vi "IP Address Facade.vi"(0 "Data In":T4="0.0.0.0", 2 "Display State In":T2, 3 "Container State":T3) -> (6 "Data Out":T4="0.0.0.0", 7 "Display State Out":T2, 8 "Action":T1)   [LabVIEW 2011, in "IP Address.xctl"]
doc: "The control takes data in the form of 4 individual unsigned bytes and automatically converts to a string representation of an IP address such as 127.0.0.1. An addition to that, the control advances the cursor to the next byte when it detects three characters, the Tab key, or the Period/Dot/Decimal key.\n\nv1.0 Copyright 2007 - Dan Press - PrimeTest Automation"
uses:
  IP Address.xctl
  IP Address Data.ctl
  <vilib>/_xctls/Container State.ctl
  IP Address State.ctl
  <vilib>/_xctls/Action.ctl
  <vilib>/_xctls/XControlSupport.lvlib
panel:
  in  "IP Address (ctl)":T5
  out "IP Address (ind)":T5
  # "."
  # "."
  # "."
  # "."
  # "."
  # "."
  # "."
  # "."
  # "."
  # "."
  # "."
  # "."
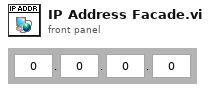
[diagram p1: front panel]
types:
  T1 = typedef "XControlSupport.lvlib/Action.ctl" = cluster{"Data Changed?":bool, "State Changed?":bool, "Action Name":string}
  T2 = typedef "IP Address.xctl/IP Address State.ctl" = cluster{"Byte":i32, "Address":cluster{"IP 0":u8, "IP 1":u8, "IP 2":u8, "IP 3":u8}}
  T3 = typedef "XControlSupport.lvlib/Container State.ctl" = cluster{"Indicator?":bool, "Run Mode?":bool, " Refnum":refnum<vi>}
  T4 = typedef "IP Address.xctl/IP Address Data.ctl" = string
  T5 = cluster{"IP 0":u8, "IP 1":u8, "IP 2":u8, "IP 3":u8}
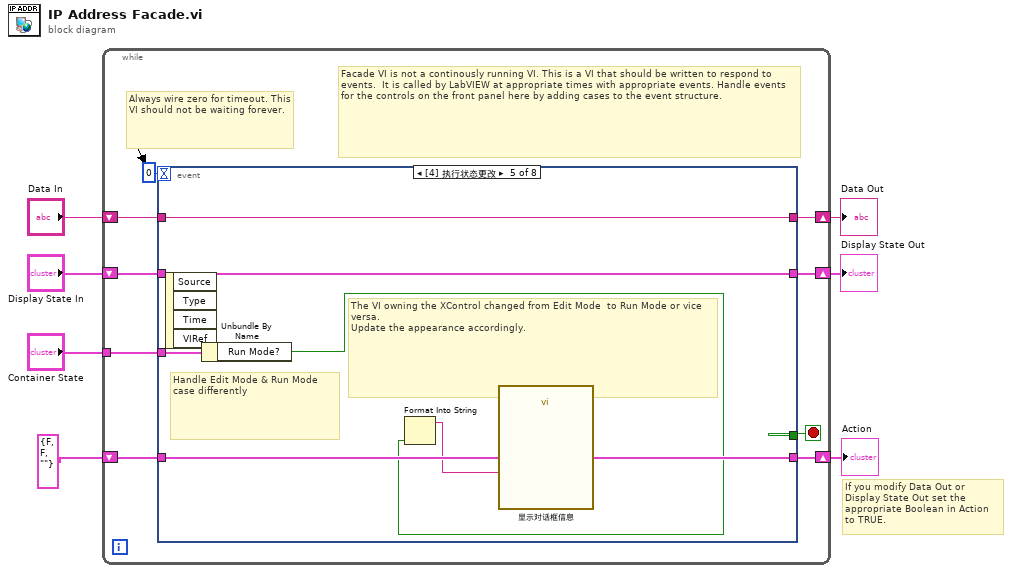
[diagram p0: block diagram]
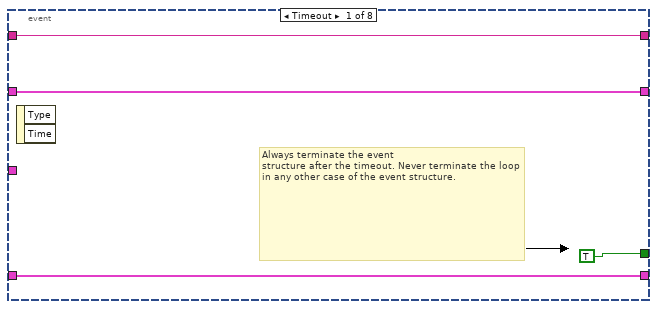
[diagram p2: hidden frame]
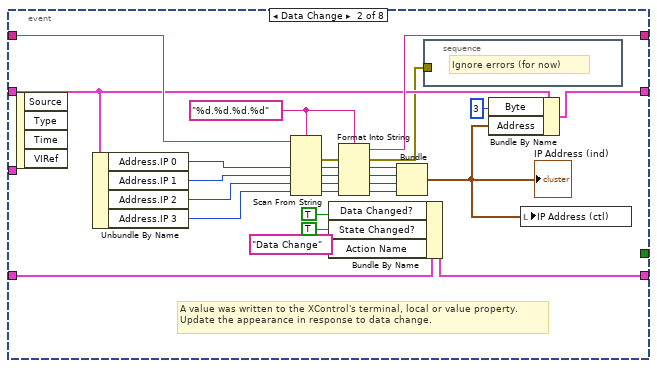
[diagram p3: hidden frame]
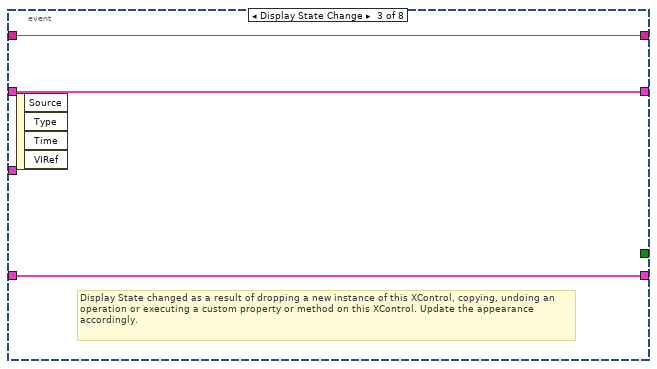
[diagram p4: hidden frame]
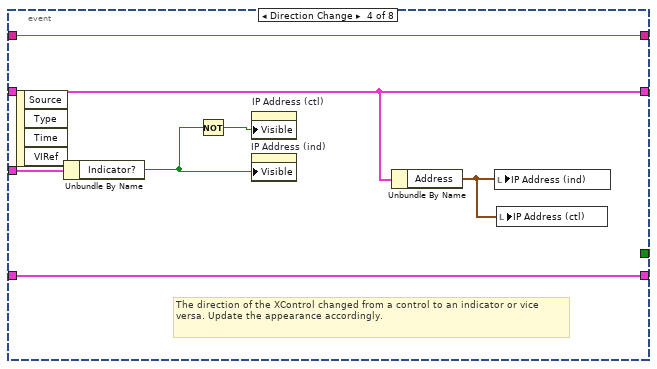
[diagram p5: hidden frame]
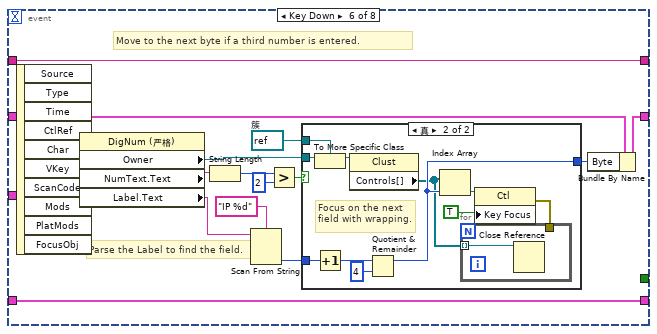
[diagram p6: hidden frame]
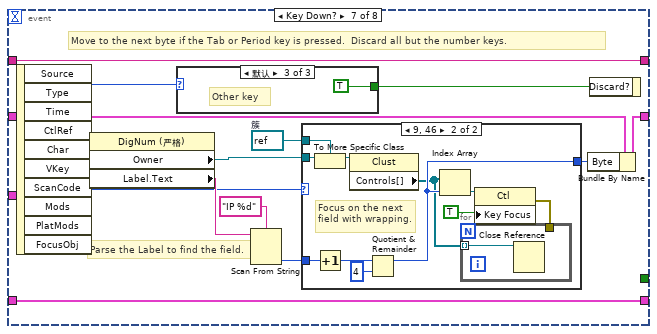
[diagram p8: hidden frame]
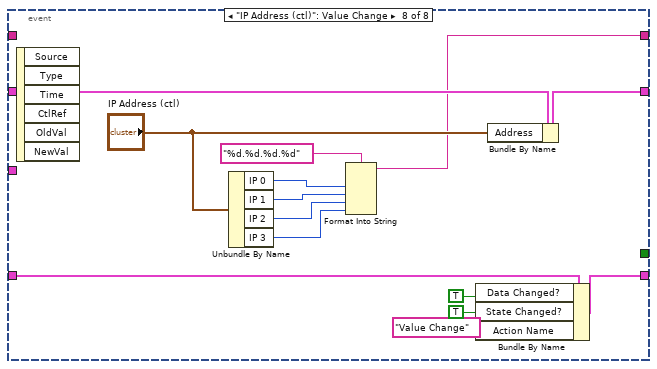
[diagram p12: hidden frame]
diagram:
  # "If you modify Data Out or\nDisplay State Out set the\nappropriate Boolean in Action\nto TRUE."
  n1 = while {
    shift-right: [w15] -> w4
    shift-left: "Display State In" -> [w16]
    tunnel: "Container State" -> [w12]
    shift-right: [w10] -> w7
    shift-left: "Data In" -> [w11]
    shift-right: [w8] -> w2
    shift-left: T1 {"Data Changed?"=FALSE, "State Changed?"=FALSE, "Action Name"=""} ("Action") -> [w9]
    stop <- w14 stop-if-true
    # "Facade VI is not a continously running VI. This is a VI that should be written to respond to events.  It is called by LabVIEW at appropriate times with appropriate events. Handle events for the controls on the front panel here by adding cases to the event structure."
    # "Always wire zero for timeout. This\nVI should not be waiting forever."
    n2 = event shown="[4] 执行状态更改" {
      selector: _ -> [_ _ _ _ _ _ _ _]
      dyn-events: _ -> [_ _ _ _ _ _ _ _]
      timeout: 0 -> [_ _ _ _ _ _ _ _]
      tunnel: w16 -> [w18 w31 w43 w47 w57 w67 w96 w127]
      tunnel: [w18 w30 w43 w47 w57 w66 w95 w126] -> w15
      tunnel: [TRUE _ _ _ _ _ _ _] -> w14
      tunnel: w12 -> [_ _ _ w52 w58 _ _ _]
      tunnel: w11 -> [w17 w33 w45 w51 w56 w73 w99 _]
      tunnel: [w17 w32 w45 w51 w56 w73 w99 w119] -> w10
      tunnel: [w19 w27 w44 w50 w55 w72 w98 w117] -> w8
      tunnel: w9 -> [w19 w28 w44 w50 w55 w72 w98 w118]
      event Timeout {
        # "Always terminate the event\nstructure after the timeout. Never terminate the loop in any other case of the event structure."
        n3 = event-data() -> ()  [unwired: 1 in, 2 out]
      }
      event Data Change {
        w34 = "%d.%d.%d.%d" ("format string")
        # "A value was written to the XControl's terminal, local or value property.\nUpdate the appearance in response to data change."
        n4 = event-data() -> ()  [unwired: 1 in, 4 out]
        n5 = Unbundle By Name(w31) -> ("Address.IP 0"=w42:u8, "Address.IP 1"=w41:u8, "Address.IP 2"=w40:u8, "Address.IP 3"=w39:u8)
        n6 = Scan From String(format string=w34, input string=w33, default 1=w42, default 2=w41, default 3=w40, default 4=w39) -> (error out=w22:errorcluster, output 1=w38:u8, output 2=w37:u8, output 3=w36:u8, output 4=w35:u8)  [unwired: 2 in, 2 out]
        n7 = Bundle By Name(cluster=w28, "Data Changed?"=TRUE, "State Changed?"=TRUE, "Action Name"="Data Change") -> (w27:T1)
        n8 = Format Into String(format string=w34, error in=w22, w38, w37, w36, w35) -> (resulting string=w32:string, error out=w21:errorcluster)  [unwired: 1 in]
        n9 = Bundle("IP 0"=w38, "IP 1"=w37, "IP 2"=w36, "IP 3"=w35) -> (w23:T5)  [unwired: 1 in]
        "IP Address (ind)" <- w23
        n10 = stacked-sequence {
          tunnel: w21 -> [_]
          frame #0 {
            # "Ignore errors (for now)"
          }
        }
        n11 = Bundle By Name(cluster=w31, "Byte"=3, "Address"=w23) -> (w30:T2)
        n12 = local write "IP Address (ctl)"(w23) -> ()
      }
      event Display State Change {
        # "Display State changed as a result of dropping a new instance of this XControl, copying, undoing an operation or executing a custom property or method on this XControl. Update the appearance accordingly."
        n13 = event-data() -> ()  [unwired: 1 in, 4 out]
      }
      event Direction Change {
        # "The direction of the XControl changed from a control to an indicator or vice versa. Update the appearance accordingly."
        n14 = event-data() -> ()  [unwired: 1 in, 4 out]
        n15 = Unbundle By Name(w52) -> ("Indicator?"=w49:bool)
        n16 = Not(x=w49) -> (.not. x?=w48:bool)
        n17 = property on="IP Address (ctl)" class="Clust (严格)"("Visible"=w48) -> ()  [unwired: 2 in, 2 out]
        n18 = property on="IP Address (ind)" class="Clust (严格)"("Visible"=w49) -> ()  [unwired: 2 in, 2 out]
        n19 = Unbundle By Name(w47) -> ("Address"=w46:T5)
        n20 = local write "IP Address (ind)"(w46) -> ()
        n21 = local write "IP Address (ctl)"(w46) -> ()
      }
      event Exec State Change {
        # "The VI owning the XControl changed from Edit Mode  to Run Mode or vice versa.\nUpdate the appearance accordingly."
        # "Handle Edit Mode & Run Mode\ncase differently"
        n22 = event-data() -> ()  [unwired: 1 in, 4 out]
        n23 = Unbundle By Name(w58) -> ("Run Mode?"=w54:bool)
        n24 = Format Into String(w54) -> (resulting string=w53:string)  [unwired: 3 in, 1 out]
        n25 = call "显示对话框信息"("Message"=w53) -> ()  [unwired: 9 in, 2 out]
      }
      event "IP Address (ctl).IP 0", "IP Address (ctl).IP 1", "IP Address (ctl).IP 2", "IP Address (ctl).IP 3": Key Down {
        w59 = refnum<vi> refnum  # 簇
        # "Move to the next byte if a third number is entered."
        # "Parse the Label to find the field."
        n26 = event-data() -> ("CtlRef"=w71:refnum<vi>)  [unwired: 1 in, 9 out]
        n27 = property class="DigNum (严格)"(reference=w71) -> ("Owner"=w60:refnum<vi>, "NumText.Text"=w70:string, "Label.Text"=w65:string)  [unwired: 1 in, 2 out]
        n28 = String Length(string=w70) -> (length=w69:i32)
        n29 = Scan From String(format string="IP %d", input string=w65) -> (output 1=w62:i32)  [unwired: 3 in, 3 out]
        n30 = Greater?(x=w69, y=2) -> (0:w63:bool)
        n31 = case shown="真" w63 {
          tunnel: w62 -> [w74 w85]
          tunnel: [w74 w79] -> w61
          tunnel: w60 -> [_ w82]
          tunnel: w59 -> [_ w80]
          frame False {
          }
          frame True {
            # "Focus on the next field with wrapping."
            n32 = To More Specific Class(target class=w80, reference=w82) -> (specific class reference=w81:refnum<vi>)  [unwired: 1 in, 1 out]
            n33 = Increment(x=w85) -> (x+1=w84:i32)
            n34 = property class="Clust"(reference=w81) -> ("Controls[]"=w77:refnum<vi>[])  [unwired: 1 in, 2 out]
            n35 = Quotient & Remainder(x=w84, y=4) -> (x-y*floor(x/y)=w79:i32)  [unwired: 1 out]
            n36 = Index Array(array=w77, index=w79) -> (element=w78:refnum<vi>)
            n37 = property class="Ctl"(reference=w78, "Key Focus"=TRUE) -> (error out=w76:errorcluster)  [unwired: 1 in, 1 out]
            n38 = for {
              tunnel: w77 -> [w86] mode=indexing
              tunnel: w76 -> [_]
              n39 = Close Reference(reference=w86) -> ()  [unwired: 1 in, 1 out]
            }
          }
        }
        n40 = Bundle By Name(cluster=w67, "Byte"=w61) -> (w66:T2)
      }
      event "IP Address (ctl).IP 0", "IP Address (ctl).IP 1", "IP Address (ctl).IP 2", "IP Address (ctl).IP 3": Key Down? {
        w89 = refnum<vi> refnum  # 簇
        # "Parse the Label to find the field."
        # "Move to the next byte if the Tab or Period key is pressed.  Discard all but the number keys."
        n41 = event-data() -> ("CtlRef"=w97:refnum<vi>, "Char"=w87:i16)  [unwired: 1 in, 8 out]
        n42 = property class="DigNum (严格)"(reference=w97) -> ("Owner"=w90:refnum<vi>, "Label.Text"=w94:string)  [unwired: 1 in, 2 out]
        n43 = case shown="默认" w87 {
          tunnel: [_ _ TRUE ("Discard?")] -> w88
          frame 48..57 {
            # "Number key"
          }
          frame 0, 8 {
            # "Backspace or delete"
          }
          frame Default {
            # "Other key"
          }
        }
        n44 = Scan From String(format string="IP %d", input string=w94) -> (output 1=w92:i32)  [unwired: 3 in, 3 out]
        n45 = case shown="9, 46" w87 {
          tunnel: w92 -> [w101 w112]
          tunnel: [w101 w106] -> w91
          tunnel: w90 -> [_ w109]
          tunnel: w89 -> [_ w107]
          frame 0, Default {
          }
          frame 9, 46 {
            # "Focus on the next field with wrapping."
            n46 = To More Specific Class(target class=w107, reference=w109) -> (specific class reference=w108:refnum<vi>)  [unwired: 1 in, 1 out]
            n47 = Increment(x=w112) -> (x+1=w111:i32)
            n48 = property class="Clust"(reference=w108) -> ("Controls[]"=w104:refnum<vi>[])  [unwired: 1 in, 2 out]
            n49 = Quotient & Remainder(x=w111, y=4) -> (x-y*floor(x/y)=w106:i32)  [unwired: 1 out]
            n50 = Index Array(array=w104, index=w106) -> (element=w105:refnum<vi>)
            n51 = property class="Ctl"(reference=w105, "Key Focus"=TRUE) -> (error out=w103:errorcluster)  [unwired: 1 in, 1 out]
            n52 = for {
              tunnel: w104 -> [w113] mode=indexing
              tunnel: w103 -> [_]
              n53 = Close Reference(reference=w113) -> ()  [unwired: 1 in, 1 out]
            }
          }
        }
        n54 = Bundle By Name(cluster=w96, "Byte"=w91) -> (w95:T2)
        n55 = event-data("Discard?"=w88) -> ()  [unwired: 1 in, 1 out]
      }
      event "IP Address (ctl)": Value Change {
        n56 = event-data() -> ()  [unwired: 1 in, 6 out]
        n57 = Unbundle By Name("IP Address (ctl)") -> ("IP 0"=w123:u8, "IP 1"=w122:u8, "IP 2"=w121:u8, "IP 3"=w120:u8)
        n58 = Format Into String(format string="%d.%d.%d.%d", w123, w122, w121, w120) -> (resulting string=w119:string)  [unwired: 2 in, 1 out]
        n59 = Bundle By Name(cluster=w118, "Data Changed?"=TRUE, "State Changed?"=TRUE ("Data Changed?"), "Action Name"="Value Change") -> (w117:T1)
        n60 = Bundle By Name(cluster=w127, "Address"="IP Address (ctl)") -> (w126:T2)
      }
    }
  }
  "Display State Out" <- w4
  "Data Out" <- w7
  "Action" <- w2
